vi "subVI_explode3array.vi"(7 "Array":dbl[](array[numeric])) -> (6 "x":dbl, 8 "y":dbl, 10 "z":dbl)   [LabVIEW 2014]
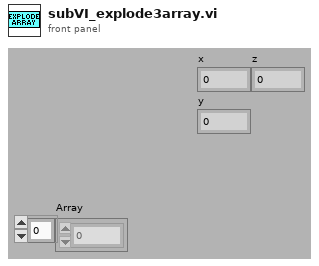
[diagram p1: front panel]
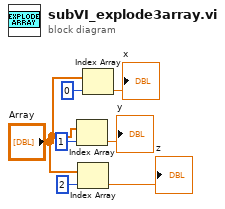
[diagram p0: block diagram]
diagram:
  n1 = Index Array(array="Array", index=1) -> (element=→"y":dbl)
  n2 = Index Array(array="Array", index=2) -> (element=→"z":dbl)
  n3 = Index Array(array="Array", index=0) -> (element=→"x":dbl)
